vi "Display Hardware Devices.vi"(8 "error in (no error)":errorcluster, 9 "Hardware Type":string, 10 "Array of Device GUIDs":string[](array[string]), 11 "Operator UI in":refnum<class "Controller UI.lvclass">) -> (0 "error out":errorcluster, 3 "Operator UI out":refnum<class "Controller UI.lvclass">)   [LabVIEW 2016, in "Controller UI.lvlib" / "Controller UI.lvclass"]
uses:
  <userlib>/Common Components/Controller UI/Controller UI.lvclass
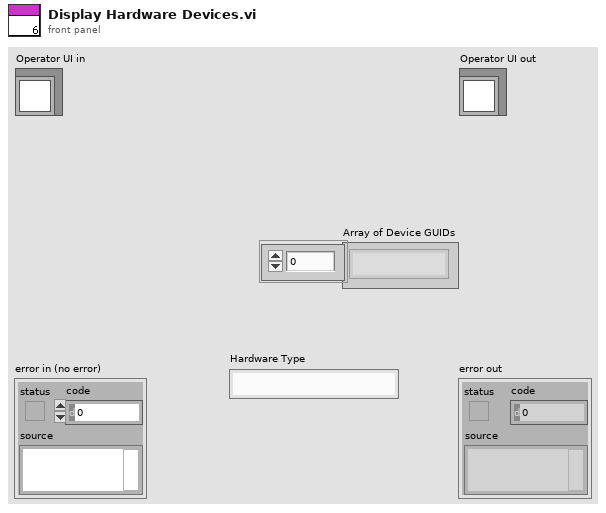
[diagram p1: front panel]
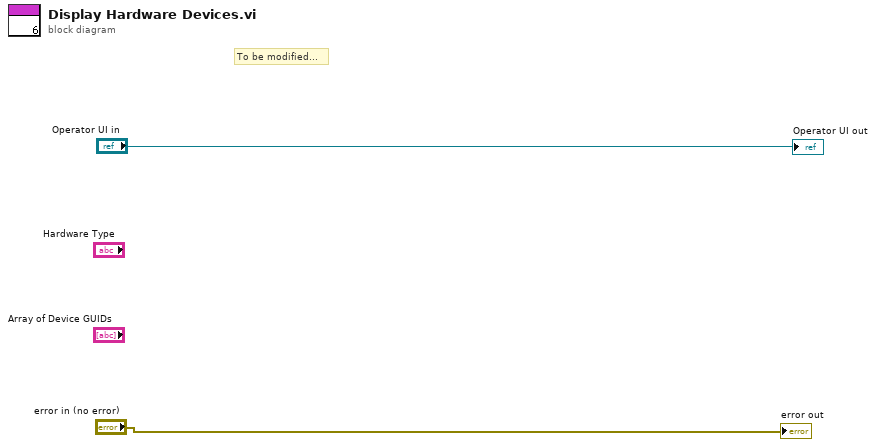
[diagram p0: block diagram]
diagram:
  # "To be modified..."
  "error out" <- "error in (no error)"
  "Operator UI out" <- "Operator UI in"
